vi "Undo.vi"(8 "error in (no error)":errorcluster, 11 "UndoObject in":refnum<class "UndoObject.lvclass">) -> (0 "error out":errorcluster, 2 "Ctrl Val.Get All":T1[](array[typedef]), 3 "UndoObject out":refnum<class "UndoObject.lvclass">, 4 "Redo Enable":bool, 6 "Undo Enable":bool)   [LabVIEW 2015, in "UndoLibrary.lvlib" / "UndoObject.lvclass"]
doc: "This VI stores the values to perform the undo action."
uses:
  UndoObject.lvclass
  Support VIs/DataClass/Controls/cluster_Control Value.ctl
  UndoObject.lvclass/UndoObject.ctl
  Support VIs/DataClass/DataObject.lvclass/DataObject.ctl
  Support VIs/DataClass/DataObject.lvclass
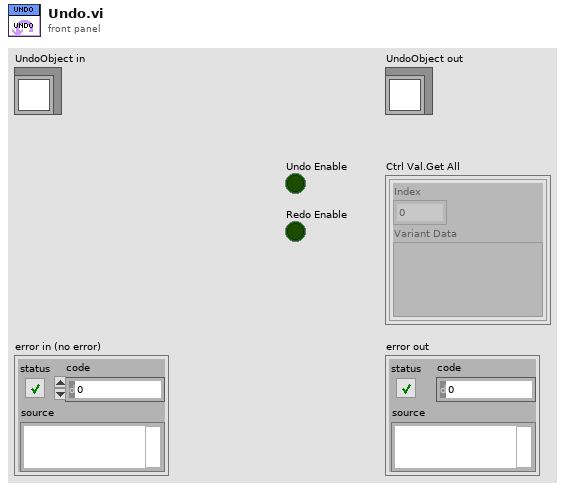
[diagram p1: front panel]
types:
  T1 = typedef "UndoLibrary.lvlib/DataObject.lvclass/cluster_Control Value.ctl" = cluster{"Index":i32, "Variant Data":variant}
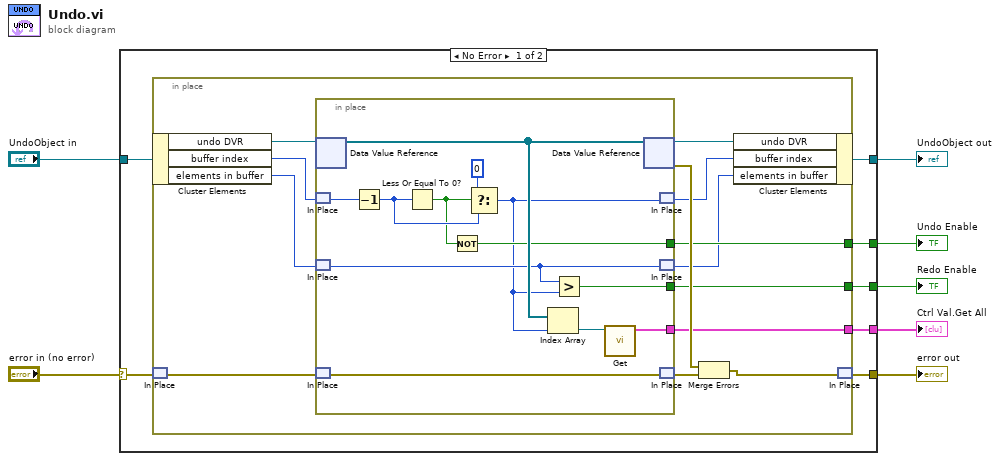
[diagram p0: block diagram]
diagram:
  n1 = case shown="No Error" "error in (no error)" {
    selector: "error in (no error)" -> [w14 w41]
    tunnel: [w13 w41] -> w7
    tunnel: "UndoObject in" -> [w12 w40]
    tunnel: [w11 w40] -> w2
    tunnel: [w10 _] -> w1
    tunnel: [w9 _] -> w5
    tunnel: [w8 _] -> w4
    frame No Error {
      n2 = in-place {
        in-place-border: [w21] -> w10
        in-place-border: [w18] -> w9
        in-place-border: [w15] -> w8
        n3 = in-place-cluster #1(w12) -> ("undo DVR"=w25:refnum<data-value>, "buffer index"=w20:i32, "elements in buffer"=w17:i32)
        n4 = in-place-match #2(w14) -> (w27:errorcluster)
        n5 = in-place {
          in-place-border: [w35] -> w18
          in-place-border: [w32] -> w21
          in-place-border: [w28] -> w15
          n6 = in-place-dvr #3(w25) -> (w36:refnum<class "DataObject.lvclass">[])  [unwired: 1 out]
          n7 = in-place-match #4(w20) -> (w31:i32)
          n8 = in-place-match #5(w17) -> (w30:i32)
          n9 = in-place-match #6(w27) -> (w34:errorcluster)
          n10 = Decrement(x=w31) -> (x-1=w38:i32)
          n11 = Less Or Equal To 0?(x=w38) -> (x <= 0?=w37:bool)
          n12 = Not(x=w37) -> (.not. x?=w35:bool)
          n13 = Select(t=0, s=w37, f=w38) -> (s? t:f=w29:i32)
          n14 = Index Array(array=w36, index=w29) -> (element=w33:refnum<class "DataObject.lvclass">)
          n15 = Greater?(x=w30, y=w29) -> (0:w28:bool)
          n16 = call "Get.vi"("DataObject in"=w33) -> ("Conrol Value[]"=w32:T1[])  [unwired: 9 in, 1 out]
          n17 = in-place-dvr #3(w36) -> (w24:refnum<data-value>, w22:errorcluster)
          n18 = in-place-match #4(w29) -> (w19:i32)
          n19 = in-place-match #5(w30) -> (w16:i32)
          n20 = in-place-match #6(w34) -> (w26:errorcluster)
        }
        n21 = Merge Errors(w22, w26) -> (w23:errorcluster)
        n22 = in-place-cluster #1("undo DVR"=w24, "buffer index"=w19, "elements in buffer"=w16) -> (w11:refnum<class "UndoObject.lvclass">)
        n23 = in-place-match #2(w23) -> (w13:errorcluster)
      }
    }
    frame Error {
    }
  }
  "error out" <- w7
  "Ctrl Val.Get All" <- w1
  "Undo Enable" <- w5
  "Redo Enable" <- w4
  "UndoObject out" <- w2
